vi "Save Keys.vi"(8 "error in (no error)":errorcluster, 11 "Configuration UI in":refnum<class "Configuration UI.lvclass">) -> (0 "error out":errorcluster, 3 "Configuration UI out":refnum<class "Configuration UI.lvclass">)   [LabVIEW 2023, in "Configuration UI.lvlib" / "Configuration UI.lvclass"]
doc: "Save all configuration key values from the editor window to the currently selected instrument to config.ini"
uses:
  Project/Configuration UI.lvclass
  Project/Configuration UI.lvclass/Configuration UI.ctl
  builds/Tools/Config.lvlibp/Config.lvclass
  builds/Engine/Engine.lvlibp/Project/Engine.lvclass
  C:/Users/Public/Documents/Development/builds/Engine/Engine.lvlibp/Project/Engine.lvclass
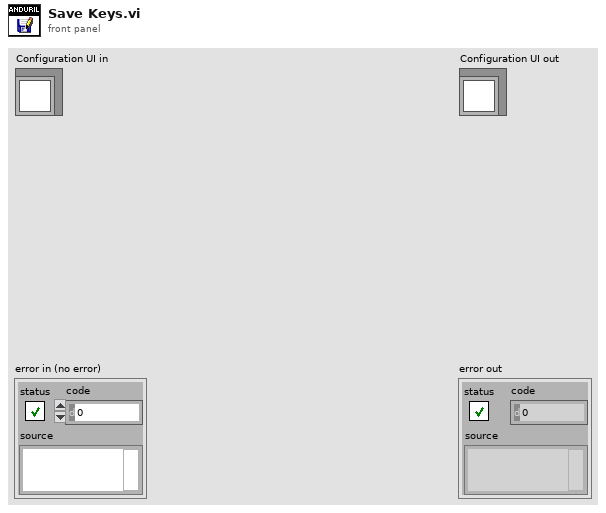
[diagram p1: front panel]
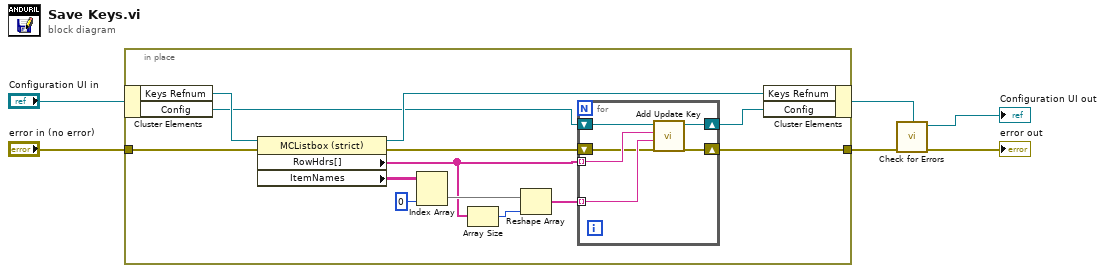
[diagram p0: block diagram]
diagram:
  n1 = in-place {
    in-place-border: "error in (no error)" -> [w10]
    in-place-border: [w7] -> w1
    n2 = in-place-cluster #1("Configuration UI in") -> ("Keys Refnum"=w19:refnum<vi>, "Config"=w11:refnum<class "Config.lvclass">)
    n3 = property class="MCListbox (strict)"(reference=w19, error in=w10) -> (reference out=w18:refnum<vi>, error out=w13:errorcluster, "RowHdrs[]"=w8:string[], "ItemNames"=w14:string[][])
    n4 = Index Array(array=w14, index (col)=0 ("disabled index (col)")) -> (element=w16:string[])  [unwired: 1 in]
    n5 = Array Size(array=w8) -> (size(s)=w17:i32)
    n6 = Reshape Array(w16, w17) -> (w9:string[])
    n7 = for {
      tunnel: w8 -> [w23] mode=indexing
      tunnel: w9 -> [w22] mode=indexing
      shift-right: [w24] -> w12
      shift-left: w11 -> [w25]
      shift-right: [w21] -> w7
      shift-left: w13 -> [w20]
      n8 = call "Add Update Key.vi"("error in"=w20, "Value"=w22, "Key"=w23, "Config in"=w25) -> ("error out"=w21:errorcluster, "Config out"=w24:refnum<class "Config.lvclass">)  [unwired: 6 in]
    }
    n9 = in-place-cluster #1("Keys Refnum"=w18, "Config"=w12) -> (w2:refnum<class "Configuration UI.lvclass">)
  }
  n10 = call "Check for Errors.vi"("error in"=w1, "Engine in"=w2) -> ("error out"=→"error out":errorcluster, "Engine out"=→"Configuration UI out":refnum<class "Configuration UI.lvclass">)  [unwired: 8 in]
